vi "Check Log Size.vi"(8 "error in":errorcluster, 10 "Data":T1[](array[typedef]), 11 "Log Producer in":refnum<class "Log Producer.lvclass">) -> (0 "error out":errorcluster, 3 "Log Producer out":refnum<class "Log Producer.lvclass">)   [LabVIEW 2020, in "AIM ARINC 664 Engine.lvlib" / "Implementation.lvlib" / "Frame Logging.lvlib"]
uses:
  Frame.ctl
  Log Producer/Log Producer.lvclass
  Frame Logging.lvlib
  Implementation.lvlib
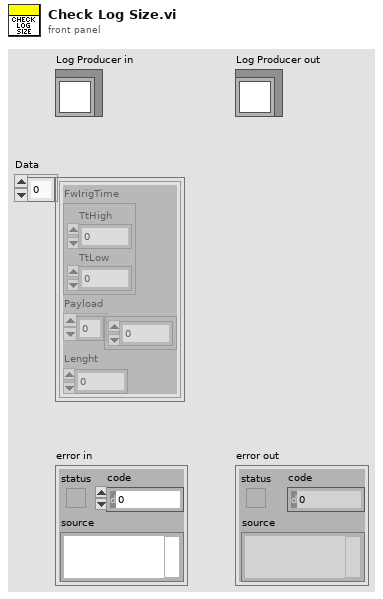
[diagram p1: front panel]
types:
  T1 = typedef "AIM ARINC 664 Engine.lvlib/Implementation.lvlib/Frame.ctl" = cluster{"FwIrigTime":cluster{"TtHigh":u32, "TtLow":u32}, "Payload":u8[], "Lenght":u32}
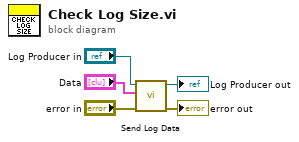
[diagram p0: block diagram]
diagram:
  n1 = call "Send Log Data.vi"("error in"="error in", "Data"="Data", "Log Producer in"="Log Producer in") -> ("error out"=→"error out":errorcluster, "Log Producer out"=→"Log Producer out":refnum<class "Log Producer.lvclass">)  [unwired: 7 in]
